vi "laplicatie.vi"() -> ()   [LabVIEW 2011]
panel:
  in  "Limita Inferioara":dbl
  in  "Limita Superioara":dbl
  out "Valoare Convertita [V]":dbl
  out "Temperatura curenta":dbl
  in  "stop 2":bool
  out "Comanda Incalzitor":bool
  out "Waveform Chart":T1(graph)
  out "Temperatura Mediie":dbl(slide) scale=0.0..100.0
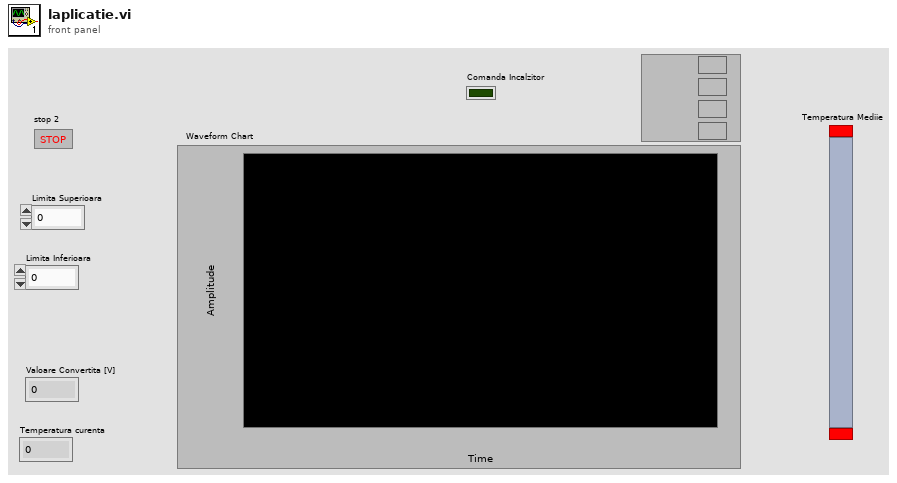
[diagram p1: front panel]
types:
  T1 = cluster{"Limita Superioara ":dbl, dbl, "Limita Inferioara":dbl, dbl}
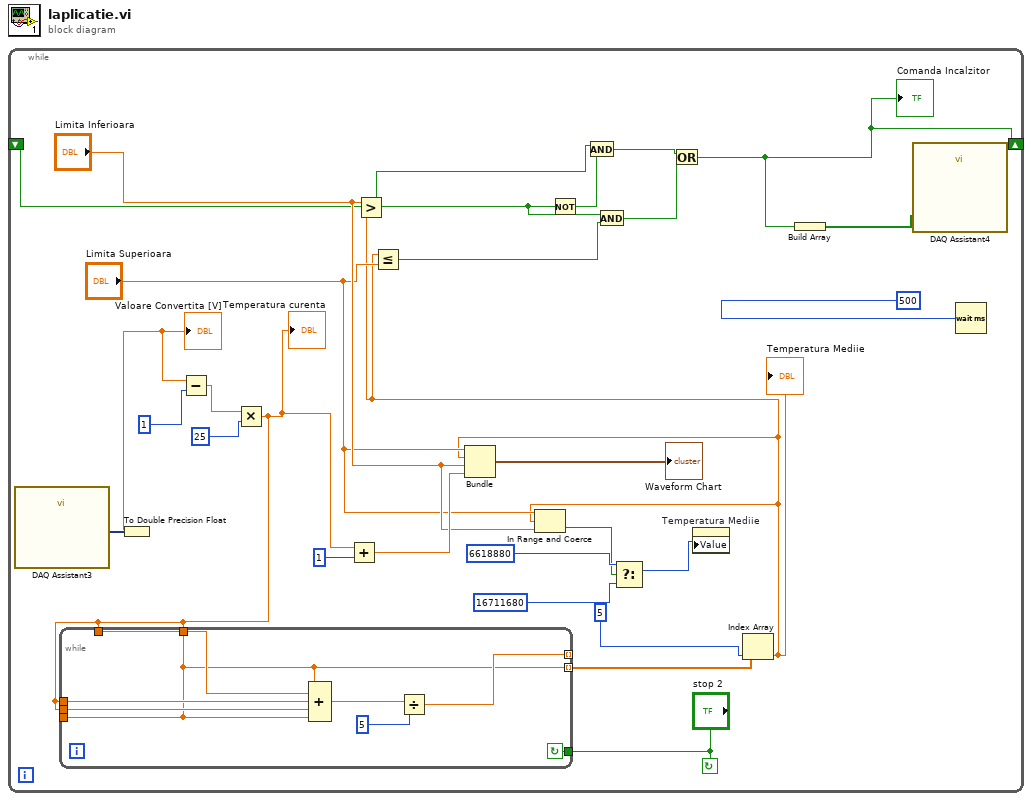
[diagram p0: block diagram]
diagram:
  n1 = while {
    shift-right: [w7] -> _
    shift-left: _ -> [w5]
    stop <- "stop 2" continue-if-true
    n2 = call "DAQ Assistant3"() -> ("data"=w25:dynamicdata)  [unwired: 17 in, 2 out]
    n3 = To Double Precision Float(number=w25) -> (double precision float=w11:dbl)
    "Valoare Convertita [V]" <- w11
    n4 = Subtract(x=w11, y=1) -> (x-y=w22:dbl)
    n5 = Multiply(x=w22, y=25) -> (x*y=w1:dbl)
    "Temperatura curenta" <- w1
    n6 = while {
      tunnel: [w34] -> _ mode=indexing
      tunnel: [w30] -> w9 mode=indexing
      tunnel: w1 -> [w33]
      tunnel: w1 -> [w32]
      tunnel: w1 -> [w31]
      tunnel: [w30] -> _
      tunnel: w1 -> [w30]
      tunnel: "stop 2" -> [w29]
      stop <- w29 continue-if-true
      n7 = Compound Arithmetic op=unknown(w30, w33, w31, w32, w30) -> (w36:dbl)
      n8 = Divide(x=w36, y=5) -> (x/y=w34:dbl)
    }
    n9 = Add(x=w1, y=1) -> (x+y=w16:dbl)
    n10 = Not(x=w5) -> (.not. x?=w4:bool)
    n11 = Index Array(array=w9, index=5) -> (element=w2:dbl)
    "Temperatura Mediie" <- w2
    n12 = Greater?(x="Limita Inferioara", y=w2) -> (0:w6:bool)
    n13 = Less Or Equal?(x=w2, y="Limita Superioara") -> (x <= y?=w21:bool)
    n14 = Bundle("Limita Superioara"="Limita Superioara", w2, "Limita Inferioara"="Limita Inferioara", w16) -> (→"Waveform Chart":T1)  [unwired: 1 in]
    n15 = In Range and Coerce(upper limit="Limita Superioara", x=w2, lower limit="Limita Inferioara") -> (In Range?=w13:bool)  [unwired: 1 out]
    n16 = And(x=w6, y=w4) -> (x .and. y?=w20:bool)
    n17 = And(x=w5, y=w21) -> (x .and. y?=w19:bool)
    n18 = Select(t=6618880, s=w13, f=16711680) -> (s? t:f=w12:i32)
    n19 = Or(x=w20, y=w19) -> (x .or. y?=w7:bool)
    "Comanda Incalzitor" <- w7
    n20 = property on="Temperatura Mediie" class="Slide (strict)"("Value"=w12) -> ()  [unwired: 2 in, 2 out]
    n21 = Build Array(w7) -> (w18:bool[])
    n22 = call "DAQ Assistant4"("data"=w18) -> ()  [unwired: 17 in, 2 out]
    n23 = Wait (ms)(milliseconds to wait=500) -> ()  [unwired: 1 out]
  }
